vi "Position and size to monitor for runtime menus.vi"(8 "error in (no error)":errorcluster, 9 "Runtime menu?":bool, 10 "Front Panel Window:Origin":cluster{"Horizontal":i16, "Vertical":i16}={"Horizontal"=0, "Vertical"=40}, 11 "vi path":path=path "C:/Projects - not VSS/Merck - Tablet Press/LV6 VIS/Merck Beta Press 100.vi") -> (0 "error out":errorcluster, 3 "monitor size":cluster{"X":i32, "Y":i32})   [LabVIEW 2013, in "GUI.lvlib"]
doc: "Positions the panel upper left corner of calling vi (from input \"vi path\") and sizes the panel to the current monitor display size."
uses:
  GUI.lvlib
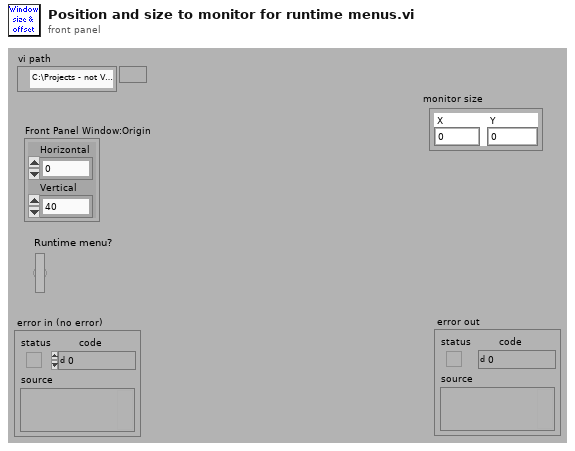
[diagram p1: front panel]
types:
  T1 = typedef "LVRectTypeDef.ctl" = cluster{"Left":i16, "Top":i16, "Right":i16, "Bottom":i16}
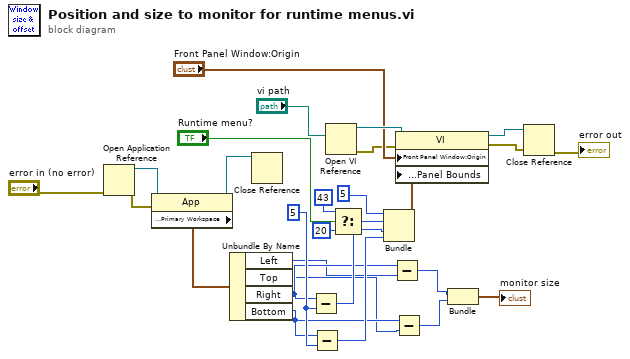
[diagram p0: block diagram]
diagram:
  w17 = i16 5 ("x")
  n1 = Open Application Reference(8:"error in (no error)") -> (0:w20:errorcluster, 3:w19:refnum<vi>)  [unwired: 3 in]
  n2 = property class="App"(reference=w19, error in=w20) -> (reference out=w13:refnum<vi>, "Display:Primary Workspace"=w18:T1)  [unwired: 1 out]
  n3 = Unbundle By Name(w18) -> ("Left"=w6:i16, "Top"=w4:i16, "Right"=w7:i16, "Bottom"=w5:i16)
  n4 = Close Reference(reference=w13) -> ()  [unwired: 1 in, 1 out]
  n5 = Subtract(x=w7, y=w17) -> (x-y=w16:i16)
  n6 = Subtract(x=w5, y=w17) -> (x-y=w15:i16)
  n7 = Open VI Reference(vi path="vi path") -> (vi reference=w28:refnum<vi>, error out=w21:errorcluster)  [unwired: 5 in]
  n8 = Select(t=i16 43 ("x"), s="Runtime menu?", f=i16 20) -> (s? t:f=w11:i16)
  n9 = Bundle("x"=i16 5, "f"=w11, w16, w15) -> (w14:cluster{"x":i16, "f":i16, i16, i16})  [unwired: 1 in]
  n10 = Subtract(x=w7, y=w6) -> (x-y=w3:i16)
  n11 = Subtract(x=w5, y=w4) -> (x-y=w2:i16)
  n12 = property class="VI"(reference=w28, error in=w21, "Front Panel Window:Origin"="Front Panel Window:Origin", "Front Panel Window:Panel Bounds"=w14) -> (reference out=w25:refnum<vi>, error out=w23:errorcluster)
  n13 = Bundle(w3, w2) -> (→"monitor size":cluster{i16, i16})  [unwired: 1 in]
  n14 = Close Reference(reference=w25, error in (no error)=w23) -> (error out=→"error out":errorcluster)
